vi "AccelFSRangeToDouble.vi"(11 "AccelFSRange":T1=enum."+/-8g") -> (3 "Double":dbl)   [LabVIEW 2016]
uses:
  AccelFSRange.ctl
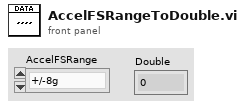
[diagram p1: front panel]
types:
  T1 = typedef "AccelFSRange.ctl" = enum16{"+/-2g", "+/-4g", "+/-8g", "+/-16g"}
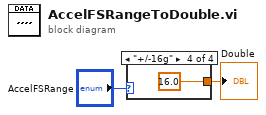
[diagram p0: block diagram]
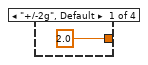
[diagram p2: hidden frame]
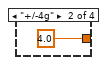
[diagram p3: hidden frame]
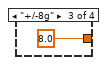
[diagram p4: hidden frame]
diagram:
  n1 = case shown="\"+/-16g\"" "AccelFSRange" {
    tunnel: [2.0 4.0 8.0 16.0] -> w1
    frame "+/-2g", Default {
    }
    frame "+/-4g" {
    }
    frame "+/-8g" {
    }
    frame "+/-16g" {
    }
  }
  "Double" <- w1
